vi "Warn_on_low_HD_space.vi"(6 "Status In":T1, 8 "HD name":string) -> (0 "Status Out":T1, 2 "free":dbl format="%.2f", 3 "used":dbl format="%.2f", 4 "error out":errorcluster, 5 "HD Size MB":dbl format="%.2f")   [LabVIEW 2010]
uses:
  Gen Trav/Multi_Run_Status.ctl
  ADAM Client/Sub VIs/ADAM Controls/Remember_value_mode.ctl
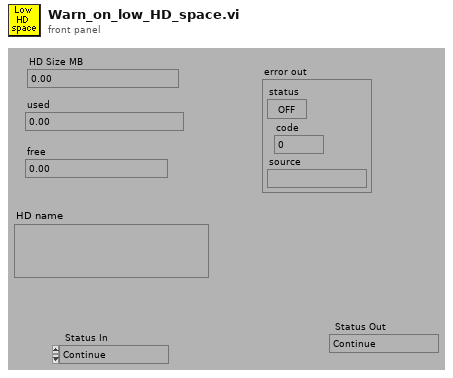
[diagram p1: front panel]
types:
  T1 = typedef "Multi_Run_Status.ctl" = enum16{"Continue", "Jump to Next Point", "Jump to Next Row", "Jump To Fall Back", "Terminate Run"}
  T2 = typedef "Remember_value_mode.ctl" = enum16{"Read only", "Read and Write"}
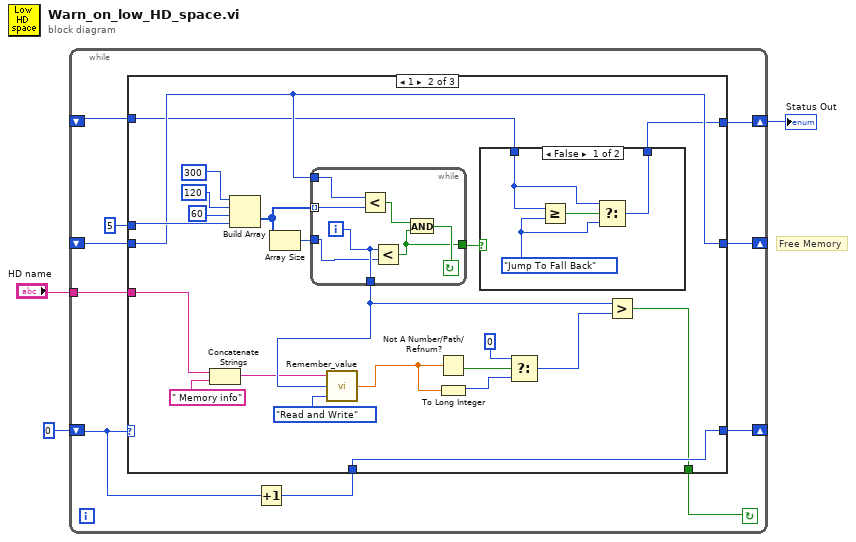
[diagram p0: block diagram]
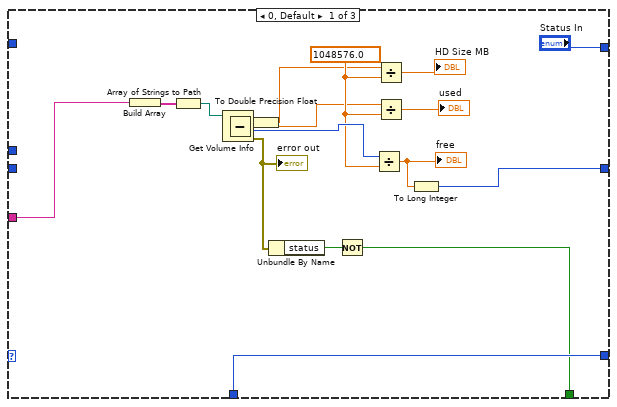
[diagram p2: hidden frame]
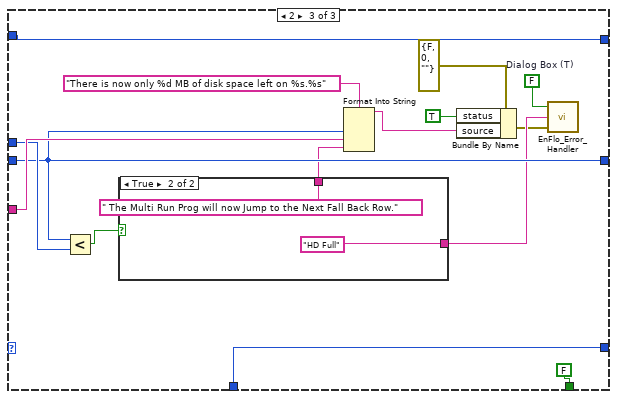
[diagram p4: hidden frame]
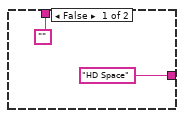
[diagram p5: hidden frame]
diagram:
  # "Free Memory"
  n1 = while {
    shift-left: _ -> [w5]
    shift-right: [w4] -> w1
    shift-left: _ -> [w7]
    shift-right: [w8] -> _
    tunnel: "HD name" -> [w9]
    shift-left: 0 -> [w13]
    shift-right: [w11] -> _
    stop <- w10 continue-if-true
    n2 = Increment(x=w13) -> (x+1=w12:i32)
    n3 = case shown="1" w13 {
      tunnel: w12 -> [w30 w47 w76]
      tunnel: [w30 w47 w76] -> w11
      tunnel: [w16 w46 FALSE] -> w10
      tunnel: w9 -> [w20 w41 w78]
      tunnel: [w19 w34 w74] -> w8
      tunnel: w7 -> [_ w34 w74]
      tunnel: 5 ("x") -> [_ w45 w75]
      tunnel: ["Status In" w32 w65] -> w4
      tunnel: w5 -> [_ w31 w65]
      frame 0, Default {
        w28 = 1048576.0 ("y")
        n4 = Build Array(w20) -> (w23:string[])
        n5 = Array of Strings to Path(0:w23) -> (2:w22:path)  [unwired: 1 out]
        n6 = Get Volume Info(11:w22) -> (0:w18:errorcluster, 1:w29:i64, 2:w14:i64)  [unwired: 1 in, 3 out]
        "error out" <- w18
        n7 = To Double Precision Float(number=w14) -> (double precision float=w27:dbl)
        n8 = Subtract(x=w27, y=w29) -> (x-y=w26:dbl)
        n9 = Unbundle By Name(w18) -> ("status"=w17:bool)
        n10 = Not(x=w17) -> (.not. x?=w16:bool)
        n11 = Divide(x=w29, y=w28) -> (x/y=w21:dbl)
        "free" <- w21
        n12 = Divide(x=w27, y=w28) -> (x/y=→"HD Size MB":dbl)
        n13 = Divide(x=w26, y=w28) -> (x/y=→"used":dbl)
        n14 = To Long Integer(number=w21) -> (32bit integer=w19:i32)
      }
      frame 1 {
        n15 = Concatenate Strings(w41, " Memory info" ("Substring")) -> (w40:string)
        n16 = Build Array(300 ("x"), 120 ("x"), 60 ("x"), w45) -> (w49:i32[])
        n17 = Array Size(array=w49) -> (size(s)=w48:i32)
        n18 = while {
          tunnel: [w53] -> w33
          tunnel: [w55] -> w43
          tunnel: w48 -> [w54]
          tunnel: w49 -> [w58] mode=indexing
          tunnel: w34 -> [w59]
          i -> [w55]
          stop <- w56 continue-if-true
          n19 = Less?(x=w59, y=w58) -> (x < y?=w57:bool)
          n20 = Less?(x=w55, y=w54) -> (x < y?=w53:bool)
          n21 = And(x=w57, y=w53) -> (x .and. y?=w56:bool)
        }
        n22 = call "Remember_value.vi"("Mode"=Remember_value_mode."Read and Write", "Input Value"=w43, "Ch name"=w40) -> ("Output Value"=w36:dbl)
        n23 = Not A Number/Path/Refnum?(number/path/refnum=w36) -> (NaN/Path/Refnum?=w39:bool)
        n24 = To Long Integer(number=w36) -> (32bit integer=w37:i32)
        n25 = case shown="False" w33 {
          tunnel: [w60 w64] -> w32
          tunnel: w31 -> [w62 w64]
          frame False {
            w61 = Multi_Run_Status."Jump To Fall Back" ("Status In")
            n26 = Greater Or Equal?(x=w62, y=w61) -> (x >= y?=w63:bool)
            n27 = Select(t=w62, s=w63, f=w61) -> (s? t:f=w60:T1)
          }
          frame True {
          }
        }
        n28 = Select(t=0, s=w39, f=w37) -> (s? t:f=w35:i32)
        n29 = Greater?(x=w43, y=w35) -> (0:w46:bool)
      }
      frame 2 {
        w68 = FALSE  # Dialog Box (T)
        n30 = Less?(x=w74, y=w75) -> (x < y?=w73:bool)
        n31 = case shown="True" w73 {
          tunnel: ["" " The Multi Run Prog will now Jump to the Next Fall Back Row." ("t")] -> w70
          tunnel: ["HD Space" "HD Full"] -> w67
          frame False {
          }
          frame True {
          }
        }
        n32 = Format Into String(format string="There is now only %d MB of disk space left on %s.%s" ("Format String"), w74, w78, w70) -> (resulting string=w69:string)  [unwired: 2 in, 1 out]
        n33 = Bundle By Name(cluster=errorcluster {"status"=FALSE, "code"=0, "source"=""} ("error in (no error)"), "status"=TRUE ("Bundle Element"), "source"=w69) -> (w66:errorcluster)
        n34 = call "EnFlo_Error_Handler.vi"("error in (no error)"=w66, "Error Type"=w67, "Dialog Box (T)"=w68) -> ()  [unwired: 3 out]
      }
    }
  }
  "Status Out" <- w1
